vi "UpdateParamsHeaders.vi"(8 "ErrorArray In":errorcluster[](array[cluster]), 9 "INIFilePaths (from Framework Data)":path[](array[path]), 10 "ParamsRef In":refnum<vi>, 11 "TypeRef":refnum<vi>) -> (0 "ErrorArray Out":errorcluster[](array[cluster]), 2 "ParamsRef Out":refnum<vi>)   [LabVIEW 2017, in "Framework.lvlib"]
uses:
  Framework.lvlib
  Init/TypeDefs/clInitParams.ctl
  <userlib>/NIST/NISTErrorLib/NISTErrorLib.lvlib
  <vilib>/Utility/config.llb/NI_LVConfig.lvlib
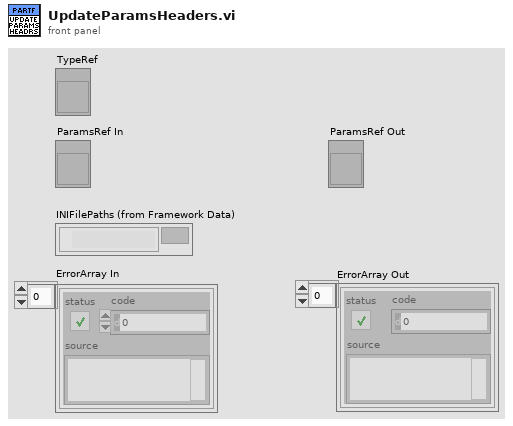
[diagram p1: front panel]
types:
  T1 = typedef "Framework.lvlib/clInitParams.ctl" = cluster{"RowHdrs":string[], "ColHdrs":string[], "DefaultParams":string[][]}
  T2 = typedef "NI_LVConfig.lvlib/Config Data RefNum.ctl" = refnum<k1>
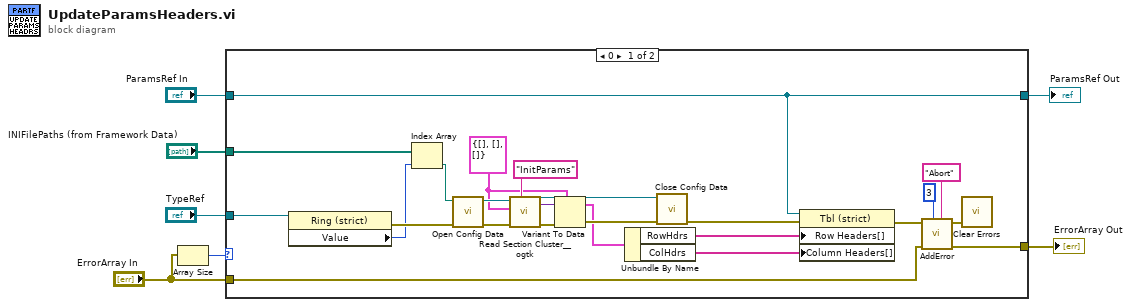
[diagram p0: block diagram]
diagram:
  n1 = Array Size(array="ErrorArray In") -> (size(s)=w7:i32)
  n2 = case shown="0" w7 {
    tunnel: "ErrorArray In" -> [w29 w33]
    tunnel: [w28 w33] -> w5
    tunnel: "TypeRef" -> [w10 _]
    tunnel: "ParamsRef In" -> [w9 w32]
    tunnel: [w9 w32] -> w2
    tunnel: "INIFilePaths (from Framework Data)" -> [w8 _]
    frame 0 {
      w21 = T1 {"RowHdrs"=[], "ColHdrs"=[], "DefaultParams"=[]} ("ParamsHdrs")
      n3 = property class="Ring (strict)"(reference=w10) -> (error out=w31:errorcluster, "Value"=w30:u16)  [unwired: 1 in, 1 out]
      n4 = Index Array(array=w8, index=w30) -> (element=w27:path)
      n5 = call <vilib>:"Open Config Data.vi"("error in (no error)"=w31, "configuration file path"=w27) -> ("error out"=w26:errorcluster, "refnum"=w25:T2)  [unwired: 7 in, 1 out]
      n6 = call <userlib>:"Read Section Cluster__ogtk.vi"("section (optional)"="InitParams", "error in (no error)"=w26, "Section Formatted Cluster Type"=w21, "refnum"=w25) -> ("error out"=w23:errorcluster, "Section Formatted Cluster"=w22:variant, "dup refnum"=w16:T2)  [unwired: 3 in, 2 out]
      n7 = Variant To Data(error in=w23, type=w21, Variant=w22) -> (data=w11:T1, error out=w17:errorcluster)
      n8 = Unbundle By Name(w11) -> ("RowHdrs"=w19:string[], "ColHdrs"=w20:string[])
      n9 = call <vilib>:"Close Config Data.vi"("error in (no error)"=w17, "refnum"=w16) -> ("error out"=w18:errorcluster)  [unwired: 8 in, 1 out]
      n10 = property on="Property Node" class="Tbl (strict)"(reference=w9, error in=w18, "Row Headers[]"=w19, "Column Headers[]"=w20) -> (error out=w12:errorcluster)  [unwired: 1 out]
      n11 = call <userlib>:"AddError.vi"("Severity"="Abort" ("String"), "Priority"=u8 3, "ErrorArray"=w29, "error in (no error)"=w12) -> ("ErrorArray"=w28:errorcluster[], "error out"=w13:errorcluster)  [unwired: 6 in]
      n12 = call <vilib>:"Clear Errors.vi"("error in (no error)"=w13) -> ()  [unwired: 5 in, 2 out]
    }
    frame 1, Default {
    }
  }
  "ErrorArray Out" <- w5
  "ParamsRef Out" <- w2
